vi "pre_scan.vi"(6 "scan_values":dbl[](array[numeric]), 8 "error in (no error)":errorcluster, 10 "config":T1={"hardware"=enum."none", "options"="", "repeats"=1, "loops"=1, "VISA"="COM7", "override_VISA"=FALSE} {"loops" min=1; "repeats" min=1}) -> (0 "error out":errorcluster)   [LabVIEW 2017]
uses:
  tools/core/var_config.ctl
  var_list.ctl
  hardware/radiant/radiant.lvlib
  hardware/sirah/sirah.lvlib
  tools/tools.lvlib
panel:
  # "Pre-scan hardware configuration"
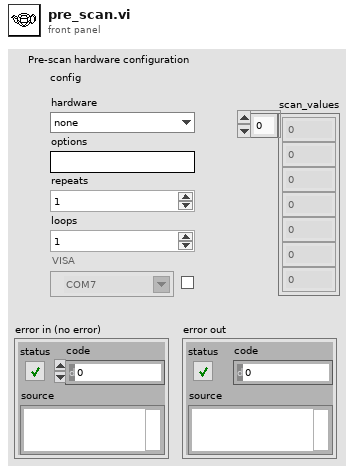
[diagram p1: front panel]
types:
  T1 = typedef "tools.lvlib/var_config.ctl" = cluster{"hardware":T2, "options":string, "repeats":i32, "loops":i32, "VISA":refnum<visa-resource-name>, "override_VISA":bool}
  T2 = typedef "var_list.ctl" = enum16{"none", "AO voltage (V)", "delay (s)", "generic", "microwaves (GHz)", "radiant (nm)", "radiant thg (nm)", "sirah (nm)", "sirah_shg (nm)", "tenma voltage (V)", "wait (s)", "wf_freq (Hz)", "wf_amp (V)", "wf_offset (V)", "wf_low_level (V)", "wf_high_level (V)", "wf_period (s)", "wf_pulse_width (s)", "wf_sample_rate (Sa/s)", "wf_multi_amp", "wf_multi_freq", "wf_arb_4chan", "WS7 setpoint (nm)"}
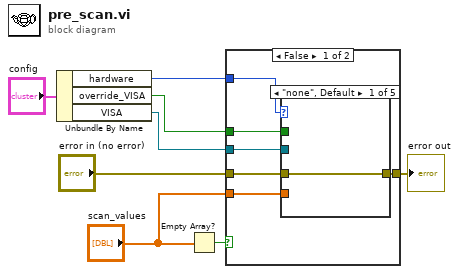
[diagram p0: block diagram]
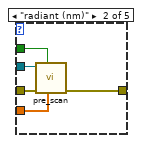
[diagram p2: hidden frame]
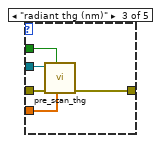
[diagram p3: hidden frame]
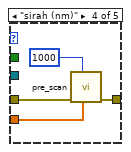
[diagram p4: hidden frame]
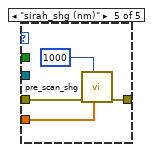
[diagram p5: hidden frame]
diagram:
  n1 = Unbundle By Name("config") -> ("hardware"=w5:T2, "override_VISA"=w3:bool, "VISA"=w4:refnum<visa-resource-name>)
  n2 = Empty Array?(array="scan_values") -> (empty?=w1:bool)
  n3 = case shown="False" w1 {
    tunnel: [w14 w34] -> w8
    tunnel: "error in (no error)" -> [w13 w34]
    tunnel: w5 -> [w12 _]
    tunnel: w4 -> [w11 _]
    tunnel: w3 -> [w10 _]
    tunnel: "scan_values" -> [w9 _]
    frame False {
      n4 = case shown="\"none\", Default" w12 {
        tunnel: [w15 w20 w25 w28 w32] -> w14
        tunnel: w13 -> [w15 w19 w24 w29 w33]
        tunnel: w11 -> [_ w18 w23 _ _]
        tunnel: w10 -> [_ w17 w22 _ _]
        tunnel: w9 -> [_ w16 w21 w27 w31]
        frame "none", Default {
        }
        frame "radiant (nm)" {
          n5 = call "pre_scan.vi"("scan_values"=w16, "override"=w17, "error in (no error)"=w19, "VISA IN"=w18) -> ("error out"=w20:errorcluster)  [unwired: 7 in]
        }
        frame "radiant thg (nm)" {
          n6 = call "pre_scan_thg.vi"("scan_values"=w21, "override"=w22, "error in (no error)"=w24, "VISA IN"=w23) -> ("error out"=w25:errorcluster)  [unwired: 7 in]
        }
        frame "sirah (nm)" {
          n7 = call "pre_scan.vi"("scan_values"=w27, "wait (ms)"=1000, "error in (no error)"=w29) -> ("error out"=w28:errorcluster)  [unwired: 8 in]
        }
        frame "sirah_shg (nm)" {
          n8 = call "pre_scan_shg.vi"("scan_values"=w31, "wait (ms)"=1000, "error in (no error)"=w33) -> ("error out"=w32:errorcluster)  [unwired: 8 in]
        }
      }
    }
    frame True {
    }
  }
  "error out" <- w8
